vi "Select Preview Channel.vi"(6 "Channel to Preview":string, 9 "Previous Selected Channel":i32, 11 "Channel Settings in":T1[](array[typedef])) -> (0 "Selected Channel":T1, 1 "Selected Channel Index":i32, 3 "Channel Settings out":T1[](array[typedef]), 5 "Selected Channel Changed?":bool)   [LabVIEW 2021, in "Settings.lvlib"]
doc: "Get the channel settings cluster and index of the channel that has the name 'Channel to Preview' in the 'Channel Settings in' array. If the index is different from the previous one, return True for 'Selected Channel Changed?'"
uses:
  Settings.lvlib
  Acquisition/Channel Settings.ctl
  Acquisition/IO Device.ctl
  Acquisition/Sensor Type.ctl
  Acquisition/Acquisition.lvlib
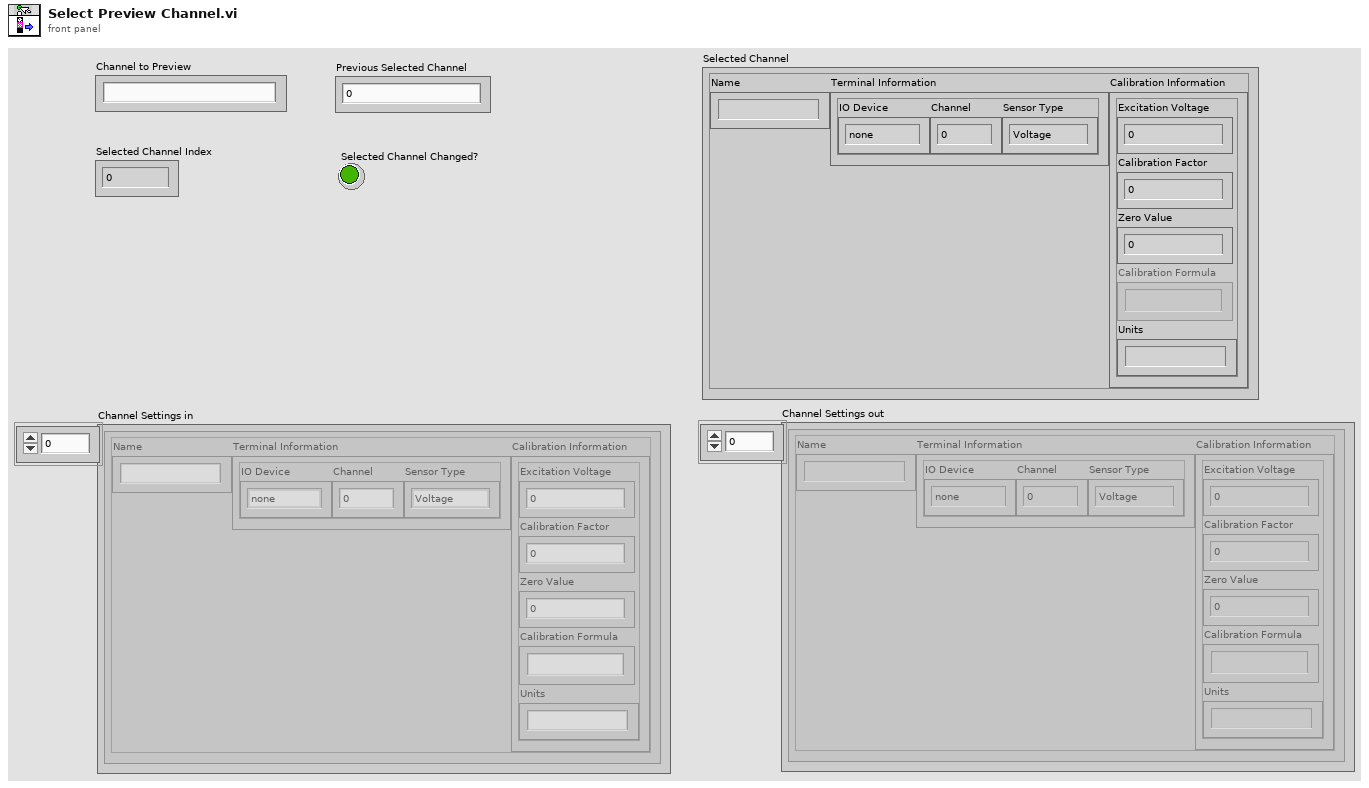
[diagram p1: front panel]
types:
  T1 = typedef "Acquisition.lvlib/Channel Settings.ctl" = cluster{"Name":string, "Terminal Information":cluster{"IO Device":T2, "Channel":i32, "Sensor Type":T3}, "Calibration Information":cluster{"Excitation Voltage":dbl, "Calibration Factor":dbl, "Zero Value":dbl, "Calibration Formula":string, "Units":string}}
  T2 = typedef "Acquisition.lvlib/IO Device.ctl" = enum16{"none", "9219", "9401"}
  T3 = typedef "Acquisition.lvlib/Sensor Type.ctl" = enum16{"Voltage", "Load", "Pressure", "Encoder"}
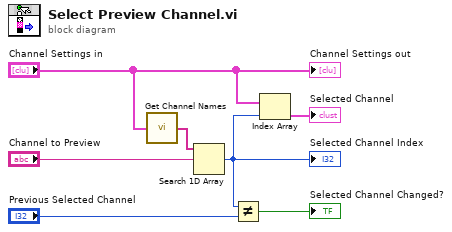
[diagram p0: block diagram]
diagram:
  n1 = call "Get Channel Names.vi"("Channel Settings"="Channel Settings in") -> ("Channel Names"=w6:string[])
  n2 = Search 1D Array(1D array=w6, element="Channel to Preview") -> (index of element=w1:i32)  [unwired: 1 in]
  "Selected Channel Index" <- w1
  n3 = Not Equal?(x=w1, y="Previous Selected Channel") -> (x != y?=→"Selected Channel Changed?":bool)
  n4 = Index Array(array="Channel Settings in", index=w1) -> (element=→"Selected Channel":T1)
  "Channel Settings out" <- "Channel Settings in"
